vi "DSF.Shared.Configuration.Transfer Group.Initialize.vi"(8 "error in (no error)":errorcluster, 10 "Transfer Group Configuration cluster":T1={"name"="", "direction"=enum."Tx", "cycle timing"={"priority"=0, "decimation"=1, "offset"=0}, "Transfers"=[], "settings"=[]}, 11 "Transfer Group Configuration in":refnum<class "VeriStand DSF.Transfer Group.Configuration.lvclass">) -> (0 "error out":errorcluster, 3 "Transfer Group Configuration out":refnum<class "VeriStand DSF.Transfer Group.Configuration.lvclass">)   [LabVIEW 2017, in "Data Sharing Framework Engine.lvlib" / "VeriStand DSF.Transfer Group.Configuration.lvclass"]
uses:
  VeriStand DSF.Transfer Group.Configuration.lvclass
  DSF Core/Built/PharLap x86/Engine/c/DSF.Engine.lvlibp/DSF Configuration API/1.0.0/Public/Controls/DSF Engine Transfer Group Configuration.ctl
  DSF Core/Built/PharLap x86/Engine/c/DSF.Engine.lvlibp/DSF Configuration API/1.0.0/Public/Controls/DSF Direction.ctl
  DSF Core/Built/PharLap x86/Engine/c/DSF.Engine.lvlibp/DSF Configuration API/1.0.0/Public/Controls/DSF Timing Info.ctl
  DSF Core/Built/PharLap x86/Engine/c/DSF.Engine.lvlibp/DSF Configuration API/1.0.0/Public/Controls/DSF Engine Transfer Configuration.ctl
  DSF Core/Built/PharLap x86/Engine/c/DSF.Engine.lvlibp/DSF Configuration API/1.0.0/Public/Controls/DSF Byte Order.ctl
  DSF Core/Built/PharLap x86/Engine/c/DSF.Engine.lvlibp/DSF Configuration API/1.0.0/Public/Controls/DSF Engine Channel Configuration.ctl
  DSF Core/Built/PharLap x86/Engine/c/DSF.Engine.lvlibp/DSF Configuration API/1.0.0/Public/Controls/DSF Data Type.ctl
  DSF Core/Built/PharLap x86/Engine/c/DSF.Engine.lvlibp/DSF Configuration API/1.0.0/Public/Controls/DSF Settings Info.ctl
  DSF Core/Built/PharLap x86/Engine/c/DSF.Engine.lvlibp/Shared/Classes/Transfer Group/DSF.Shared.Configuration.Transfer Group.lvclass
  DSF Core/Built/PharLap x86/Engine/c/DSF.Engine.lvlibp/DSF Configuration API/1.0.0/DSF Configuration API.lvlib
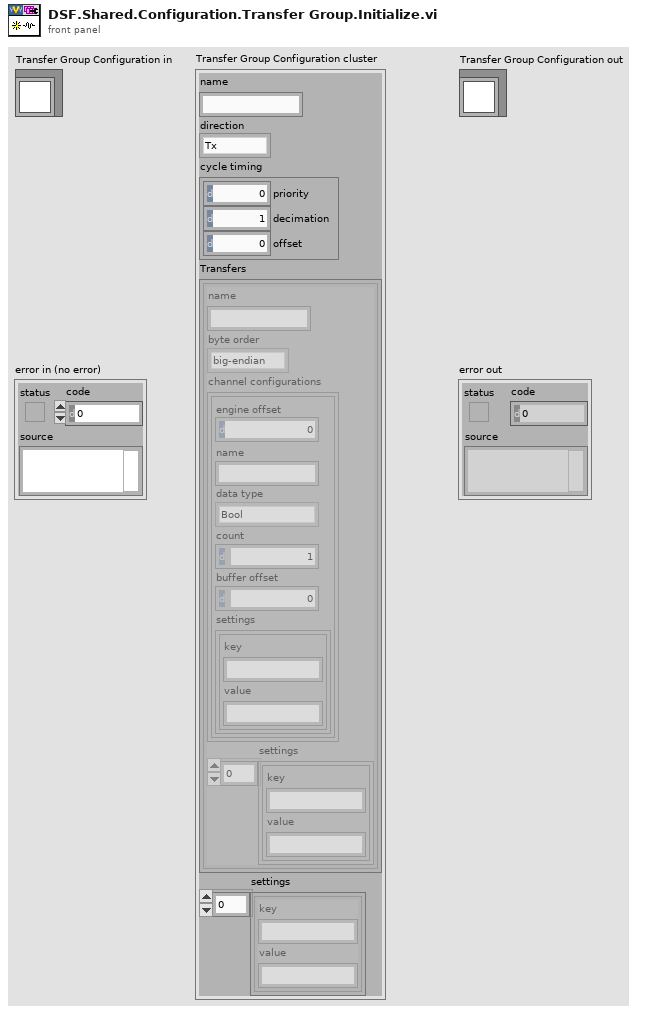
[diagram p1: front panel]
types:
  T1 = typedef "DSF.Engine.lvlibp/DSF Configuration API.lvlib/DSF Engine Transfer Group Configuration.ctl" = cluster{"name":string, "direction":T2, "cycle timing":T3, "Transfers":T4[], "settings":T8}
  T2 = typedef "DSF.Engine.lvlibp/DSF Configuration API.lvlib/DSF Direction.ctl" = enum8{"Tx", "Rx"}
  T3 = typedef "DSF.Engine.lvlibp/DSF Configuration API.lvlib/DSF Timing Info.ctl" = cluster{"priority":u64, "decimation":u64, "offset":u64}
  T4 = typedef "DSF.Engine.lvlibp/DSF Configuration API.lvlib/DSF Engine Transfer Configuration.ctl" = cluster{"name":string, "byte order":T5, "channel configurations":T6[], "settings":T8}
  T5 = typedef "DSF.Engine.lvlibp/DSF Configuration API.lvlib/DSF Byte Order.ctl" = enum8{"big-endian", "little-endian"}
  T6 = typedef "DSF.Engine.lvlibp/DSF Configuration API.lvlib/DSF Engine Channel Configuration.ctl" = cluster{"engine offset":u64, "name":string, "data type":T7, "count":u64, "buffer offset":u64, "settings":T8}
  T7 = typedef "DSF.Engine.lvlibp/DSF Configuration API.lvlib/DSF Data Type.ctl" = enum8{"Bool", "SGL", "DBL", "I8", "I16", "I32", "I64", "U8", "U16", "U32", "U64"}
  T8 = typedef "DSF.Engine.lvlibp/DSF Configuration API.lvlib/DSF Settings Info.ctl" = cluster{"key":string, "value":string}[]
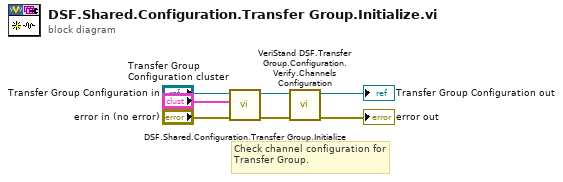
[diagram p0: block diagram]
diagram:
  # "Check channel configuration for Transfer Group."
  n1 = call-parent "DSF.Shared.Configuration.Transfer Group.Initialize.vi"("error in (no error)"="error in (no error)", "Transfer Group Configuration cluster"="Transfer Group Configuration cluster", "Transfer Group Configuration in"="Transfer Group Configuration in") -> ("error out"=w3:errorcluster, "Transfer Group Configuration"=w4:refnum<class "VeriStand DSF.Transfer Group.Configuration.lvclass">)  [unwired: 7 in]
  n2 = call "VeriStand DSF.Transfer Group.Configuration.Verify.Channels Configuration.vi"("error in (no error)"=w3, "Transfer Group Configuration in"=w4) -> ("error out"=→"error out":errorcluster, "Transfer Group Configuration out"=→"Transfer Group Configuration out":refnum<class "VeriStand DSF.Transfer Group.Configuration.lvclass">)  [unwired: 8 in]
